vi "Draw Line Segment.vi"(4 "pen":T1={"Width"=2, "Style"=enum."Solid"}, 6 "color":u32(colorbox)=11841024, 9 "End":cluster{"x":i16, "y":i16}={"x"=201, "y"=72}, 10 "Start":cluster{"x":i16, "y":i16}={"x"=201, "y"=72}, 11 "Picture In (New)":picture) -> (3 "Picture":picture)   [LabVIEW 2020, in "App.lvlib" / "MazeUI.lvclass"]
uses:
  MazeUI.lvclass
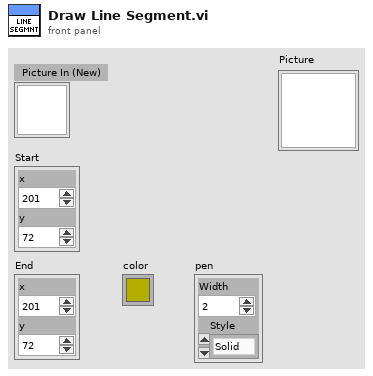
[diagram p1: front panel]
types:
  T1 = cluster{"Width":u16, "Style":enum32{"Solid", "Dash", "Dot", "DashDot", "DashDotDot"}}
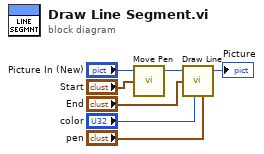
[diagram p0: block diagram]
diagram:
  n1 = call <vilib>:"Move Pen.vi"("new position"="Start", "picture"="Picture In (New)") -> ("new picture"=w6:picture)  [unwired: 3 in]
  n2 = call <vilib>:"Draw Line.vi"("picture"=w6, "end point"="End", "color(black)"="color", "pen"="pen") -> ("new picture"=→"Picture":picture)  [unwired: 5 in]
